vi "CloseDetector.vi"(0 "Averaging Size":i32=100, 1 "Initialize? (F)":bool, 2 "MaxVelosity":u16, 7 "ENCODER":i32) -> (4 "stop":bool)   [LabVIEW 2019]
uses:
  <userlib>/_MGI/1D Array/MGI Average Type Enum.ctl
  <userlib>/_MGI/1D Array/MGI Running Average/MGI Running Average(DBL).vi
panel:
  out "enable stop":bool
  out "Waveform Chart":dbl(graph)
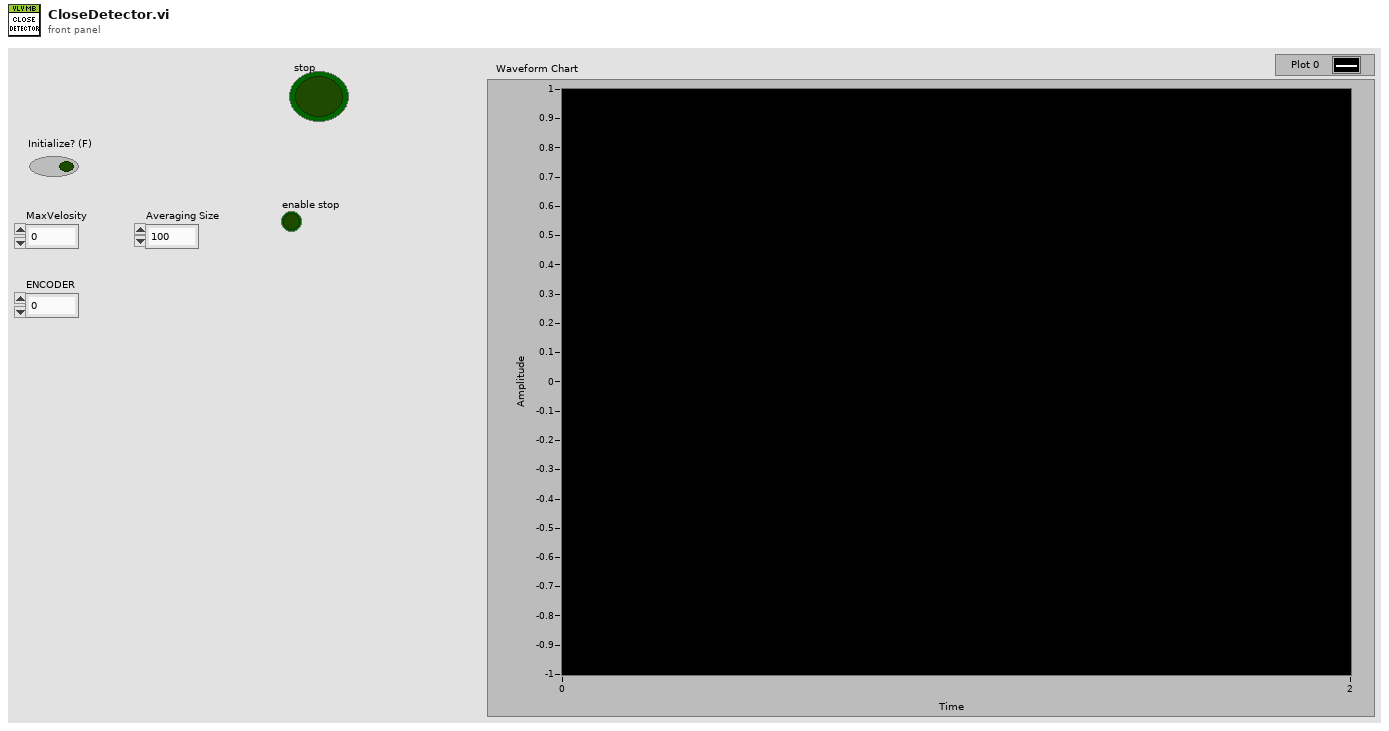
[diagram p1: front panel]
types:
  T1 = typedef "MGI Average Type Enum.ctl" = enum16{"Finite Impulse Response", "Infinite Impulse Response"}
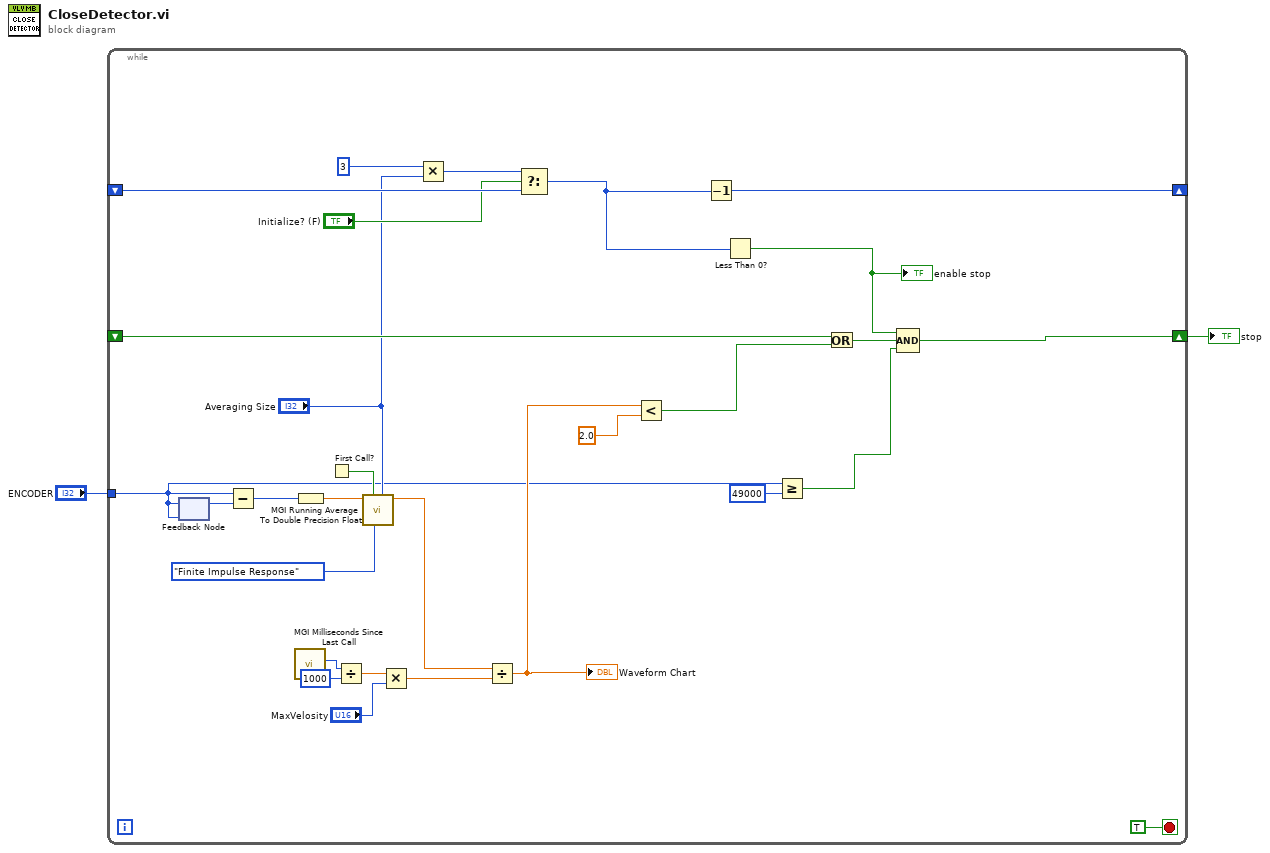
[diagram p0: block diagram]
diagram:
  n1 = while {
    tunnel: "ENCODER" -> [w5]
    shift-right: [w11] -> w1
    shift-left: _ -> [w20]
    shift-right: [w17] -> _
    shift-left: _ -> [w15]
    stop <- TRUE stop-if-true
    n2 = feedback #1(w5) -> (w31:i32)
    n3 = feedback-in #1(w5) -> ()
    n4 = Subtract(x=w5, y=w31) -> (x-y=w30:i32)
    n5 = call <userlib>:"MGI Milliseconds Since Last Call.vi"() -> ("ms"=w23:u32)  [unwired: 6 in, 1 out]
    n6 = To Double Precision Float(number=w30) -> (double precision float=w29:dbl)
    n7 = First Call?() -> (First Call?: T/F=w9:bool)
    n8 = Divide(x=w23, y=u32 1000) -> (x/y=w25:dbl)
    n9 = call-poly <userlib>:"MGI Running Average.vi"("Averaging Size"="Averaging Size", "Average Type(FIR)"=MGI_Average_Type_Enum."Finite Impulse Response", "Initialize? (F)"=w9, "Value"=w29) -> ("Average"=w22:dbl)  [unwired: 7 in]
    n10 = Multiply(x=w25, y="MaxVelosity") -> (x*y=w24:dbl)
    n11 = Multiply(x=3, y="Averaging Size") -> (x*y=w14:i32)
    n12 = Divide(x=w22, y=w24) -> (x/y=w6:dbl)
    "Waveform Chart" <- w6
    n13 = Select(t=w14, s="Initialize? (F)", f=w15) -> (s? t:f=w16:i32)
    n14 = Less?(x=w6, y=2.0) -> (x < y?=w19:bool)
    n15 = Decrement(x=w16) -> (x-1=w17:i32)
    n16 = Less Than 0?(x=w16) -> (x < 0?=w10:bool)
    "enable stop" <- w10
    n17 = Greater Or Equal?(x=w5, y=49000) -> (x >= y?=w3:bool)
    n18 = Or(x=w20, y=w19) -> (x .or. y?=w12:bool)
    n19 = Compound Arithmetic op=AND(w10, w12, w3) -> (w11:bool)
  }
  "stop" <- w1
